vi "ComputeAntennaCenter.vi"(10 "TestZT":cluster{"Z mm":dbl, "Horizontal T deg":dbl}, 11 "Motion64.ini Position Array":T1(array[cluster])) -> (0 "error out":errorcluster, 3 "Solution Vector, y and x":dbl[](array[numeric]))   [LabVIEW 2019]
doc: "Based on the four corners of the Motion64.ini file, compute the X, Y of the center of the antenna."
panel:
  out "error":i32
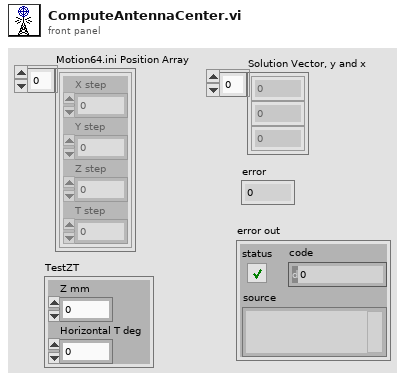
[diagram p1: front panel]
types:
  T1 = cluster{"X step":dbl, "Y step":dbl, "Z step":dbl, "T step":dbl}[]
  T2 = cluster{"X step":dbl, "Y step":dbl, "Z step":dbl, "T step":dbl}
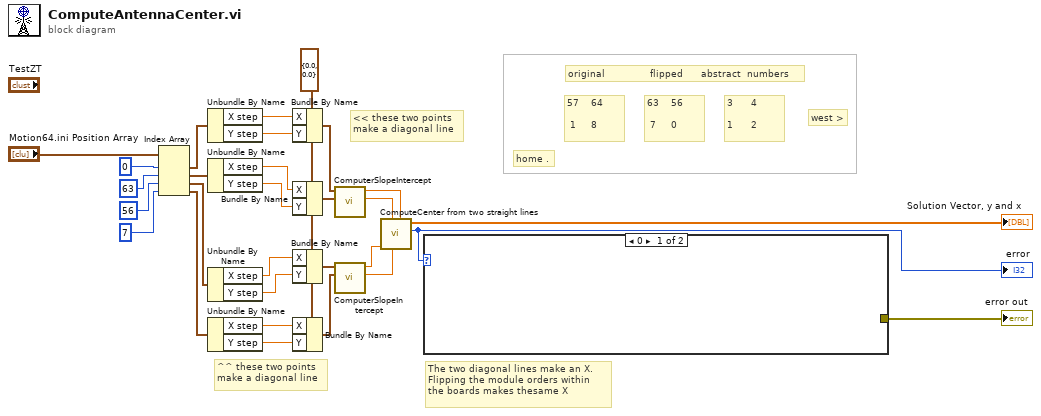
[diagram p0: block diagram]
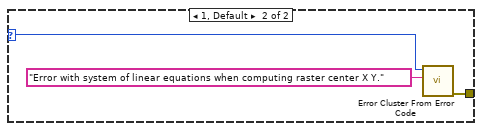
[diagram p2: hidden frame]
diagram:
  w13 = cluster{"X":sgl, "Y":sgl} {"X"=0.0, "Y"=0.0} ("Point1 (Pixels)")
  # "The two diagonal lines make an X.\nFlipping the module orders within \nthe boards makes thesame X"
  # "^^ these two points\nmake a diagonal line"
  # "<< these two points\nmake a diagonal line"
  # "original               flipped      abstract  numbers"
  # "west >"
  # "home ."
  # "3      4\n\n1      2"
  # "63    56\n\n 7     0"
  # "57    64\n\n 1     8"
  n1 = Index Array(array="Motion64.ini Position Array", index #1=0 ("index"), index #2=63 ("index"), index #3=56 ("index"), index #4=7 ("index")) -> (element #1=w22:T2, element #2=w25:T2, element #3=w24:T2, element #4=w23:T2)
  n2 = Unbundle By Name(w22) -> ("X step"=w18:dbl, "Y step"=w17:dbl)
  n3 = Unbundle By Name(w25) -> ("X step"=w21:dbl, "Y step"=w16:dbl)
  n4 = Unbundle By Name(w24) -> ("X step"=w15:dbl, "Y step"=w20:dbl)
  n5 = Unbundle By Name(w23) -> ("X step"=w19:dbl, "Y step"=w14:dbl)
  n6 = Bundle By Name(cluster=w13, "X"=w18, "Y"=w17) -> (w11:cluster{"X":sgl, "Y":sgl})
  n7 = Bundle By Name(cluster=w13, "X"=w21, "Y"=w16) -> (w10:cluster{"X":sgl, "Y":sgl})
  n8 = Bundle By Name(cluster=w13, "X"=w15, "Y"=w20) -> (w9:cluster{"X":sgl, "Y":sgl})
  n9 = Bundle By Name(cluster=w13, "X"=w19, "Y"=w14) -> (w8:cluster{"X":sgl, "Y":sgl})
  n10 = call "ComputerSlopeIntercept.vi"("Point2 (Pixels)"=w10, "Point1 (Pixels)"=w11) -> ("intercept"=w6:dbl, "slope"=w7:dbl)  [unwired: 4 in, 4 out]
  n11 = call "ComputerSlopeIntercept.vi"("Point2 (Pixels)"=w8, "Point1 (Pixels)"=w9) -> ("intercept"=w4:dbl, "slope"=w5:dbl)  [unwired: 4 in, 4 out]
  n12 = call "ComputeCenter from two straight lines.vi"("slope 2"=w7, "intercept"=w4, "intercept 2"=w6, "slope"=w5) -> ("error"=w2:i32, "Solution Vector"=→"Solution Vector, y and x":dbl[])  [unwired: 6 in]
  "error" <- w2
  n13 = case shown="0" w2 {
    selector: w2 -> [_ w30]
    tunnel: [_ w31] -> w1
    frame 0 {
    }
    frame 1, Default {
      n14 = call <vilib>:"Error Cluster From Error Code.vi"("error message (\"\")"="Error with system of linear equations when computing raster center X Y." ("error message (\"\")"), "error code (0)"=w30) -> ("error out"=w31:errorcluster)  [unwired: 7 in]
    }
  }
  "error out" <- w1
